vi "GetPhysicalChannelsSubVI.vi"(8 "error in (no error)":errorcluster) -> (0 "error out":errorcluster, 3 "Physical Channels":string[][](array[string]))   [LabVIEW 2017]
uses:
  <userlib>/_OpenG.lib/array/array.llb/Search 1D Array (String)__ogtk.vi
  <userlib>/_OpenG.lib/array/array.llb/Delete Elements from 1D Array (String)__ogtk.vi
  <resource>/objmgr/daqmx.rc
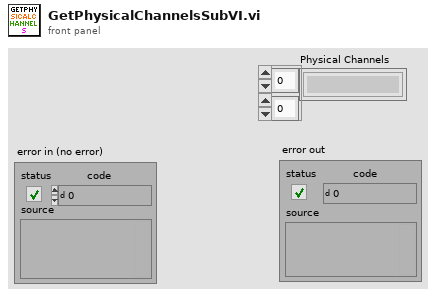
[diagram p1: front panel]
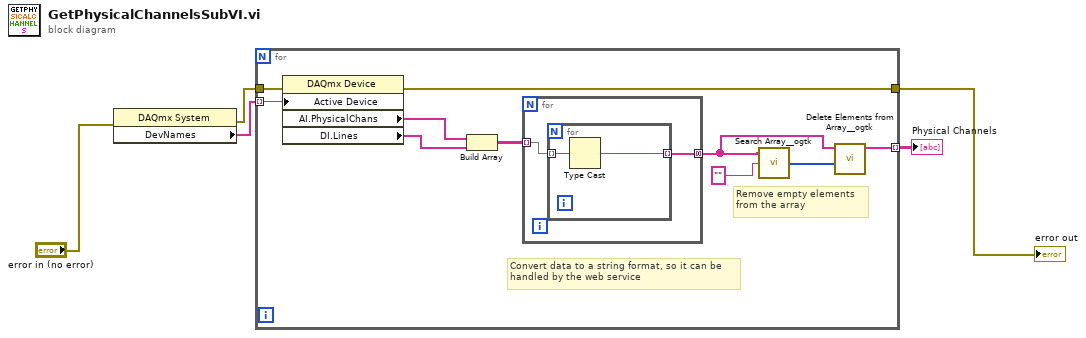
[diagram p0: block diagram]
diagram:
  n1 = property class="DAQmx System"(error in="error in (no error)") -> (error out=w3:errorcluster, "DevNames"=w5:tag[])  [unwired: 1 in, 1 out]
  n2 = for {
    tunnel: w5 -> [w15] mode=indexing
    tunnel: w3 -> [w14]
    tunnel: [w13] -> w2
    tunnel: [w6] -> w1 mode=indexing
    # "Remove empty elements\nfrom the array"
    # "Convert data to a string format, so it can be\nhandled by the web service"
    n3 = property class="DAQmx Device"(error in=w14, "Active Device"=w15) -> (error out=w13:errorcluster, "AI.PhysicalChans"=w12:tag[], "DI.Lines"=w10:tag[])  [unwired: 1 in, 1 out]
    n4 = Build Array(w12, w10) -> (w11:tag[][])
    n5 = for {
      tunnel: w11 -> [w17] mode=indexing
      tunnel: [w16] -> w8 mode=concatenating
      n6 = for {
        tunnel: w17 -> [w19] mode=indexing
        tunnel: [w18] -> w16 mode=indexing
        n7 = Type Cast(x=w19) -> (*(type *) &x=w18:string)  [unwired: 1 in]
      }
    }
    n8 = call-poly <userlib>:"Search Array__ogtk.vi"("Array"=w8, "Element Data"="") -> ("Indices of Elements"=w7:i32[])  [unwired: 7 in]
    n9 = call-poly <userlib>:"Delete Elements from Array__ogtk.vi"("indices"=w7, "array"=w8) -> ("array w/ subset deleted"=w6:string[])  [unwired: 8 in, 1 out]
  }
  "error out" <- w2
  "Physical Channels" <- w1
